vi "ABOUT_FILE.vi"() -> ()   [LabVIEW 2019]
panel:
  out "error out 2":errorcluster
  in  "Path 2":path
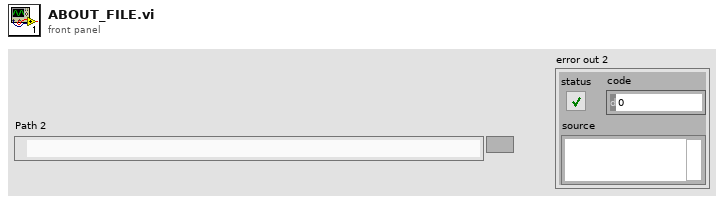
[diagram p1: front panel]
types:
  T1 = enum16{"open", "replace", "create", "open or create", "replace or create", "replace or create with confirmation"}
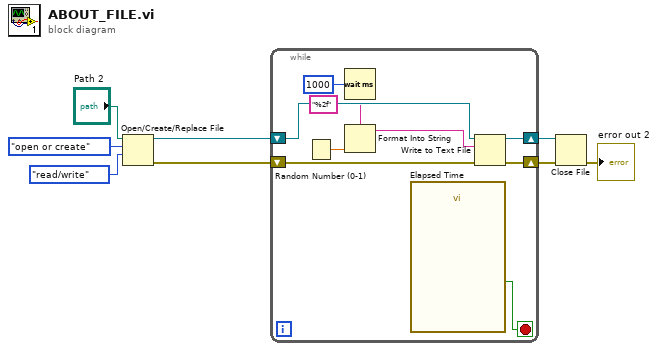
[diagram p0: block diagram]
diagram:
  n1 = Open/Create/Replace File(file path (use dialog)="Path 2", operation (0:open)=T1."open or create", access (0:read/write)=enum16{"read/write", "read-only", "write-only"}."read/write") -> (refnum out=w5:refnum<file>, error out=w4:errorcluster)  [unwired: 3 in, 1 out]
  n2 = while {
    shift-right: [w13] -> w3
    shift-left: w5 -> [w15]
    shift-right: [w12] -> w2
    shift-left: w4 -> [w14]
    stop <- w10 stop-if-true
    n3 = Random Number (0-1)() -> (number: 0 to 1=w17:dbl)
    n4 = Wait (ms)(milliseconds to wait=u32 1000) -> ()  [unwired: 1 out]
    n5 = Format Into String(format string="%2f", w17) -> (resulting string=w16:string)  [unwired: 2 in, 1 out]
    n6 = call "Elapsed Time"() -> ("Time has Elapsed"=w10:bool)  [unwired: 12 in, 7 out]
    n7 = Write to Text File(file (use dialog)=w15, text=w16, error in=w14) -> (refnum out=w13:refnum<file>, error out=w12:errorcluster)  [unwired: 1 in, 1 out]
  }
  n8 = Close File(refnum=w3, error in=w2) -> (error out=→"error out 2":errorcluster)  [unwired: 1 out]
